vi "Front Panel.vi"(11 "GUI in":refnum<class "GUI.lvclass">) -> ()   [LabVIEW 2018, in "GUI.lvclass"]
uses:
  GUI.lvclass
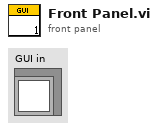
[diagram p1: front panel]
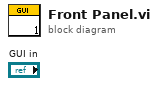
[diagram p0: block diagram]
diagram:
